vi "InitializeTimeCluster3.vi"() -> (0 "[OUT] Colocalization Properties":T1)   [LabVIEW 2013]
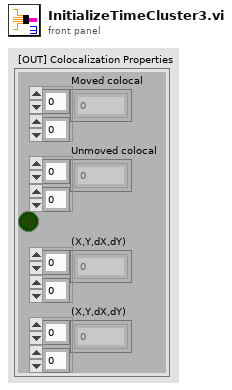
[diagram p1: front panel]
types:
  T1 = cluster{"Moved colocal":dbl[][], "Unmoved colocal":dbl[][], bool, "(X,Y,dX,dY)":dbl[][], "(X,Y,dX,dY)":dbl[][]}
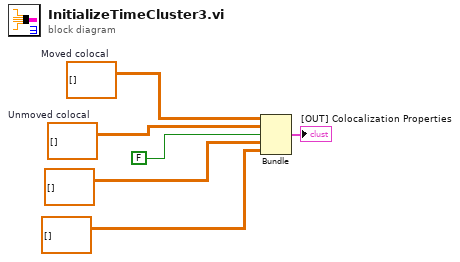
[diagram p0: block diagram]
diagram:
  w6 = dbl[][] []  # Moved colocal
  w5 = dbl[][] []  # Unmoved colocal
  n1 = Bundle("Moved colocal"=w6, "Unmoved colocal"=w5, FALSE, "(X,Y,dX,dY)"=dbl[][] [], "(X,Y,dX,dY)"=dbl[][] []) -> (→"[OUT] Colocalization Properties":T1)  [unwired: 1 in]
